vi "DeleteTag.vi"(8 "error in (no error)":errorcluster, 11 "ClassDataTree in":refnum<class "ClassDataTree.lvclass">) -> (0 "error out":errorcluster, 3 "ClassDataTree out":refnum<class "ClassDataTree.lvclass">)   [LabVIEW 2016, in "ClassDataTree.lvclass"]
uses:
  ClassDataTree.lvclass
  ClassDataTree.lvclass/ClassDataTree.ctl
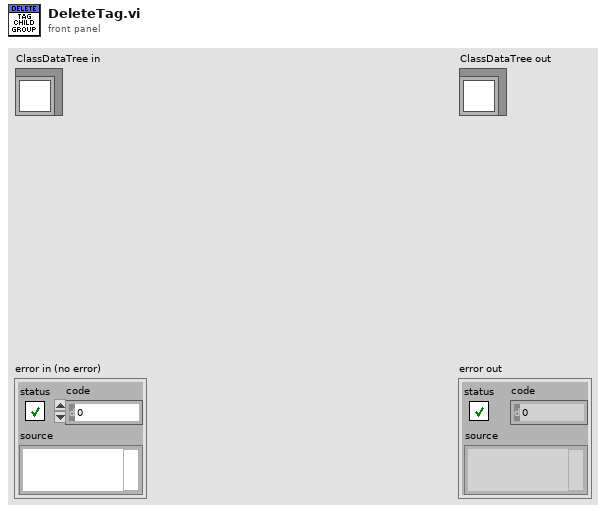
[diagram p1: front panel]
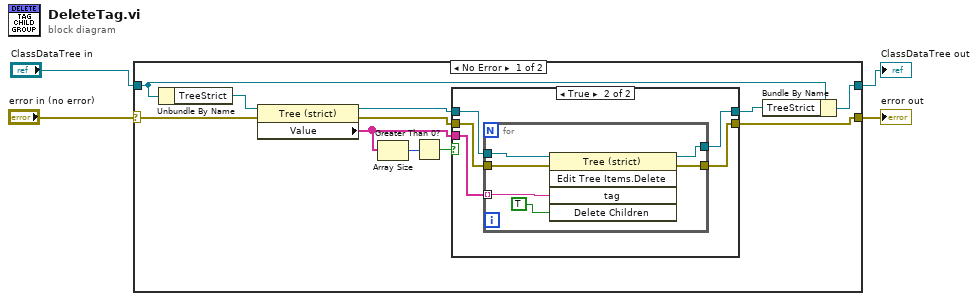
[diagram p0: block diagram]
diagram:
  n1 = case shown="No Error" "error in (no error)" {
    selector: "error in (no error)" -> [w12 w30]
    tunnel: [w8 w30] -> w2
    tunnel: [w10 w29] -> w1
    tunnel: "ClassDataTree in" -> [w11 w29]
    frame No Error {
      n2 = Unbundle By Name(w11) -> ("TreeStrict"=w15:refnum<vi>)
      n3 = property class="Tree (strict)"(reference=w15, error in=w12) -> (reference out=w14:refnum<vi>, error out=w13:errorcluster, "Value"=w7:string[])
      n4 = Array Size(array=w7) -> (size(s)=w6:i32)
      n5 = Greater Than 0?(x=w6) -> (x > 0?=w5:bool)
      n6 = case shown="True" w5 {
        tunnel: w14 -> [w17 w22]
        tunnel: w7 -> [_ w21]
        tunnel: w13 -> [w16 w20]
        tunnel: [w17 w19] -> w9
        tunnel: [w16 w18] -> w8
        frame False {
        }
        frame True {
          n7 = for {
            tunnel: w22 -> [w28]
            tunnel: w21 -> [w25] mode=indexing
            tunnel: w20 -> [w26]
            tunnel: [w24] -> w19
            tunnel: [w23] -> w18
            n8 = invoke class="Tree (strict)" method="Edit Tree Items.Delete"(reference=w28, error in=w26, "tag"=w25, "Delete Children"=TRUE ("Delete Children?")) -> (reference out=w24:refnum<vi>, error out=w23:errorcluster)  [unwired: 1 in, 3 out]
          }
        }
      }
      n9 = Bundle By Name(cluster=w11, "TreeStrict"=w9) -> (w10:refnum<class "ClassDataTree.lvclass">)
    }
    frame Error {
    }
  }
  "error out" <- w2
  "ClassDataTree out" <- w1
